vi "FindAnalyzer.vi"(8 "error in (no error)":errorcluster) -> (0 "error out":errorcluster, 1 "IsFound":bool, 2 "Information":string)   [LabVIEW 2014]
uses:
  USBAnalyzerEllisysDll.dll
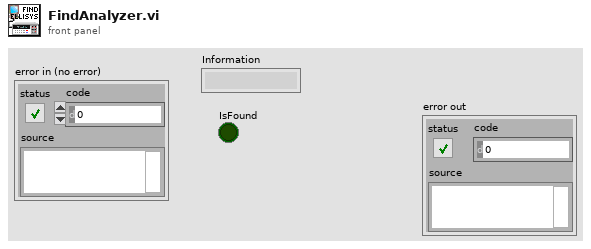
[diagram p1: front panel]
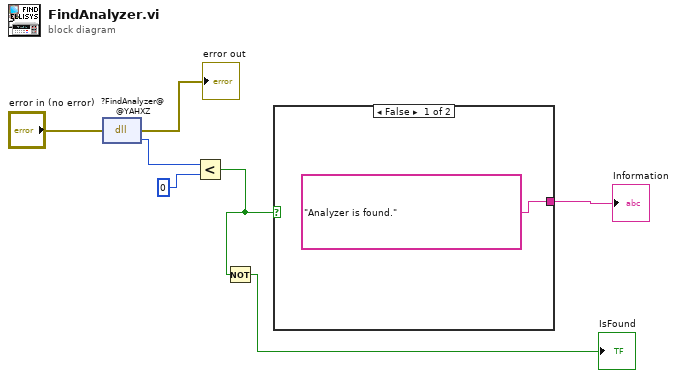
[diagram p0: block diagram]
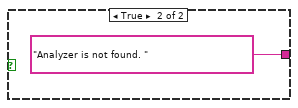
[diagram p2: hidden frame]
diagram:
  n1 = dll-call lib="PTH2labs CUsersMichał\tDocumentsEllisysAnalyzerUSBAnalyzerEllisysDllDebugUSBAnalyzerEllisysDll.dll" fn="?FindAnalyzer@@YAHXZ"(error in="error in (no error)") -> (error out=→"error out":errorcluster, "return type"=w7:i32)  [unwired: 2 in, 1 out]
  n2 = Less?(x=w7, y=0) -> (x < y?=w4:bool)
  n3 = Not(x=w4) -> (.not. x?=→"IsFound":bool)
  n4 = case shown="False" w4 {
    tunnel: ["Analyzer is found." "Analyzer is not found. "] -> w5
    frame False {
    }
    frame True {
    }
  }
  "Information" <- w5
